vi "Size.vi"   [LabVIEW 2020, in "image.lvlib"]
uses:
  image.lvlib
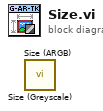
[diagram p0: block diagram]
diagram:
  n1 = call "Size (Greyscale).vi"() -> ()  [unwired: 9 in, 3 out]
  n2 = call "Size (ARGB).vi"() -> ()  [unwired: 9 in, 3 out]
